vi "Heartbeat_Create.vi"(8 "Error In":errorcluster, 11 "reference in":refnum<class "Heartbeat.lvclass">) -> (0 "Error Out":errorcluster, 3 "reference out":refnum<class "Heartbeat.lvclass">)   [LabVIEW 2024, in "CANopen Master.lvlib" / "Heartbeat.lvclass"]
uses:
  Heartbeat.lvclass
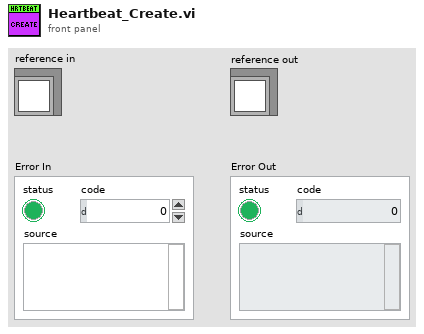
[diagram p1: front panel]
types:
  T1 = typedef "CANopen Master.lvlib/Heartbeat.lvclass/ObjectAttributes.ctl" = cluster{"Heartbeats":map{u8, cluster{"Period":u16, "Timeout":u16, "Last Beat":refnum<class "Time Stamp.lvclass">}}}
  T2 = map{u8, cluster{"Period":u16, "Timeout":u16, "Last Beat":refnum<class "Time Stamp.lvclass">}}
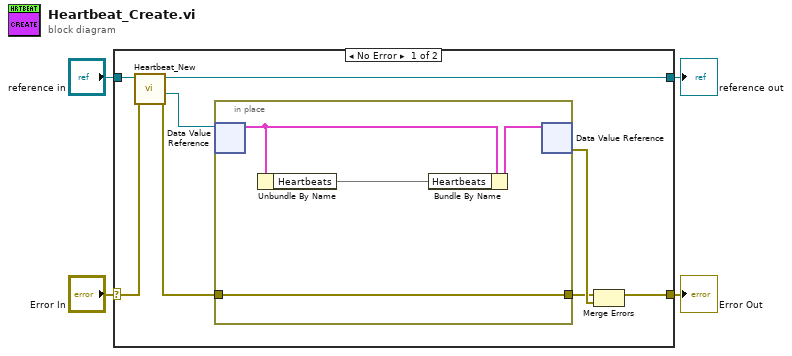
[diagram p0: block diagram]
diagram:
  n1 = case shown="No Error" "Error In" {
    selector: "Error In" -> [w11 w18]
    tunnel: [w5 w18] -> w3
    tunnel: "reference in" -> [w12 w17]
    tunnel: [w10 w17] -> w1
    frame No Error {
      n2 = call "Heartbeat_New.vi"("Error In"=w11, "reference in"=w12) -> ("Error Out"=w7:errorcluster, "DVRRefOut"=w8:refnum<data-value>, "reference out"=w10:refnum<class "Heartbeat.lvclass">)  [unwired: 6 in, 1 out]
      n3 = in-place {
        in-place-border: w7 -> [w14]
        in-place-border: [w14] -> w6
        n4 = in-place-dvr #1(w8) -> (w15:T1)  [unwired: 1 out]
        n5 = Unbundle By Name(w15) -> ("Heartbeats"=w13:T2)
        n6 = Bundle By Name(cluster=w15, "Heartbeats"=w13) -> (w16:T1)
        n7 = in-place-dvr #1(w16) -> (w9:errorcluster)  [unwired: 1 out]
      }
      n8 = Merge Errors(w6, w9) -> (w5:errorcluster)
    }
    frame Error {
      # "VI-TechBaseTemplate_Simple_4x4x4"
    }
  }
  "Error Out" <- w3
  "reference out" <- w1
